vi "deeplabv3_onnx_camera.vi"() -> ()   [LabVIEW 2018]
uses:
  <vilib>/addons/VIRobotics/opencv_yiku/ctls/ColorConversionCodes.ctl
  <vilib>/addons/VIRobotics/opencv_yiku/Mat/Mat_32F/Mat_32F.lvclass
  C:/Program Files/National Instruments/LabVIEW 2018/vi.lib/addons/VIRobotics/opencv_yiku/Mat/Mat/Mat.lvclass
  <vilib>/addons/VIRobotics/opencv_yiku/Mat/Mat_8U/Mat_8U.lvclass
  <vilib>/addons/VIRobotics/opencv_yiku/Mat/Mat/Mat_length.vi
  <vilib>/addons/VIRobotics/onnx/Session/Get_Result_float.vi
  <vilib>/addons/VIRobotics/opencv_yiku/Mat/Mat/Mat_release.vi
  <vilib>/addons/VIRobotics/opencv_yiku/opencv_yiku.lvlib
  <vilib>/addons/VIRobotics/opencv_yiku/Mat/Mat/Mat.lvclass
  <vilib>/addons/VIRobotics/onnx/Session/Session.lvclass
  <vilib>/addons/VIRobotics/opencv_yiku/Cap/Cap.lvclass
panel:
  out "x-y":u32
  out "classes":cluster{"Color":u32, "name":string}[](array[cluster])
  in  "type":enum16{"CPU", "CUDA", "TensorRT"}(ring)=enum."TensorRT"
  in  "stop":bool
  out "mask":picture
  out "原始图像":picture
  out "合成的图像":picture
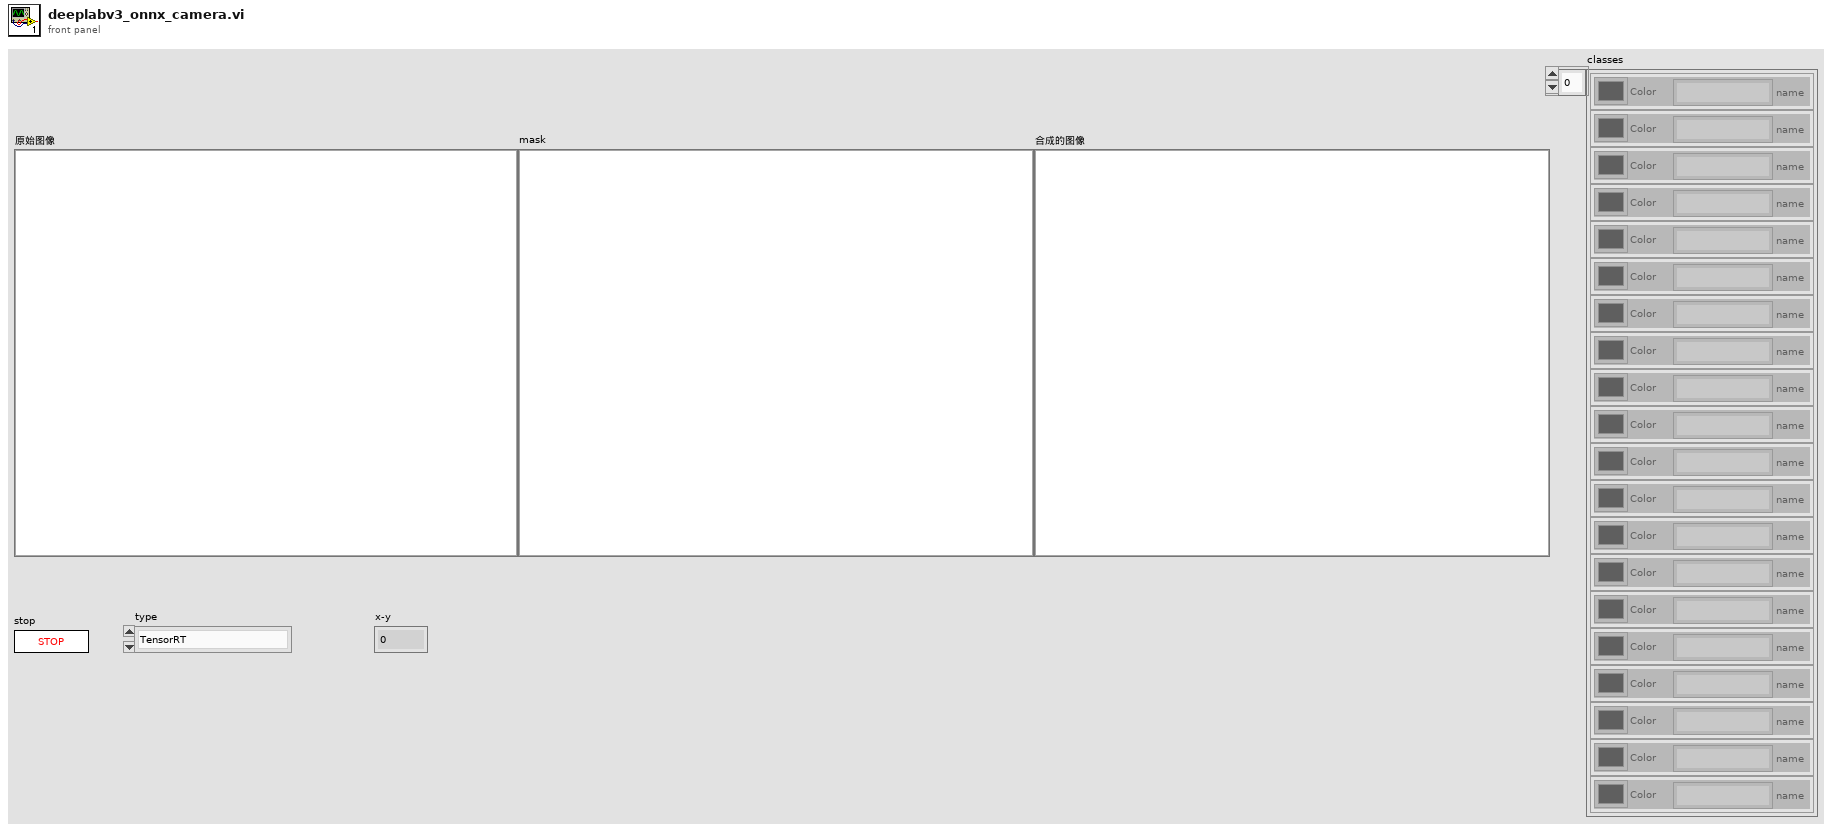
[diagram p1: front panel]
types:
  T1 = typedef "opencv_yiku.lvlib/ColorConversionCodes.ctl" = enum32{"COLOR_BGR2BGRA", "COLOR_BGRA2BGR", "COLOR_BGR2RGBA", "COLOR_RGBA2BGR", "COLOR_BGR2RGB", "COLOR_BGRA2RGBA", "COLOR_BGR2GRAY", "COLOR_RGB2GRAY", "COLOR_GRAY2BGR", "COLOR_GRAY2BGRA", "COLOR_BGRA2GRAY", "COLOR_RGBA2GRAY", "COLOR_BGR2BGR565", "COLOR_RGB2BGR565", "COLOR_BGR5652BGR", "COLOR_BGR5652RGB", "COLOR_BGRA2BGR565", "COLOR_RGBA2BGR565", "COLOR_BGR5652BGRA", "COLOR_BGR5652RGBA", "COLOR_GRAY2BGR565", "COLOR_BGR5652GRAY", "COLOR_BGR2BGR555", "COLOR_RGB2BGR555", "COLOR_BGR5552BGR", "COLOR_BGR5552RGB", "COLOR_BGRA2BGR555", "COLOR_RGBA2BGR555", "COLOR_BGR5552BGRA", "COLOR_BGR5552RGBA", "COLOR_GRAY2BGR555", "COLOR_BGR5552GRAY", "COLOR_BGR2XYZ", "COLOR_RGB2XYZ", "COLOR_XYZ2BGR", "COLOR_XYZ2RGB", "COLOR_BGR2YCrCb", "COLOR_RGB2YCrCb", "COLOR_YCrCb2BGR", "COLOR_YCrCb2RGB", "COLOR_BGR2HSV", "COLOR_RGB2HSV", "42", "43", "COLOR_BGR2Lab", "COLOR_RGB2Lab"}
  T2 = cluster{"height":i32, "width":i32, "channels":i32, "pointer":u64}
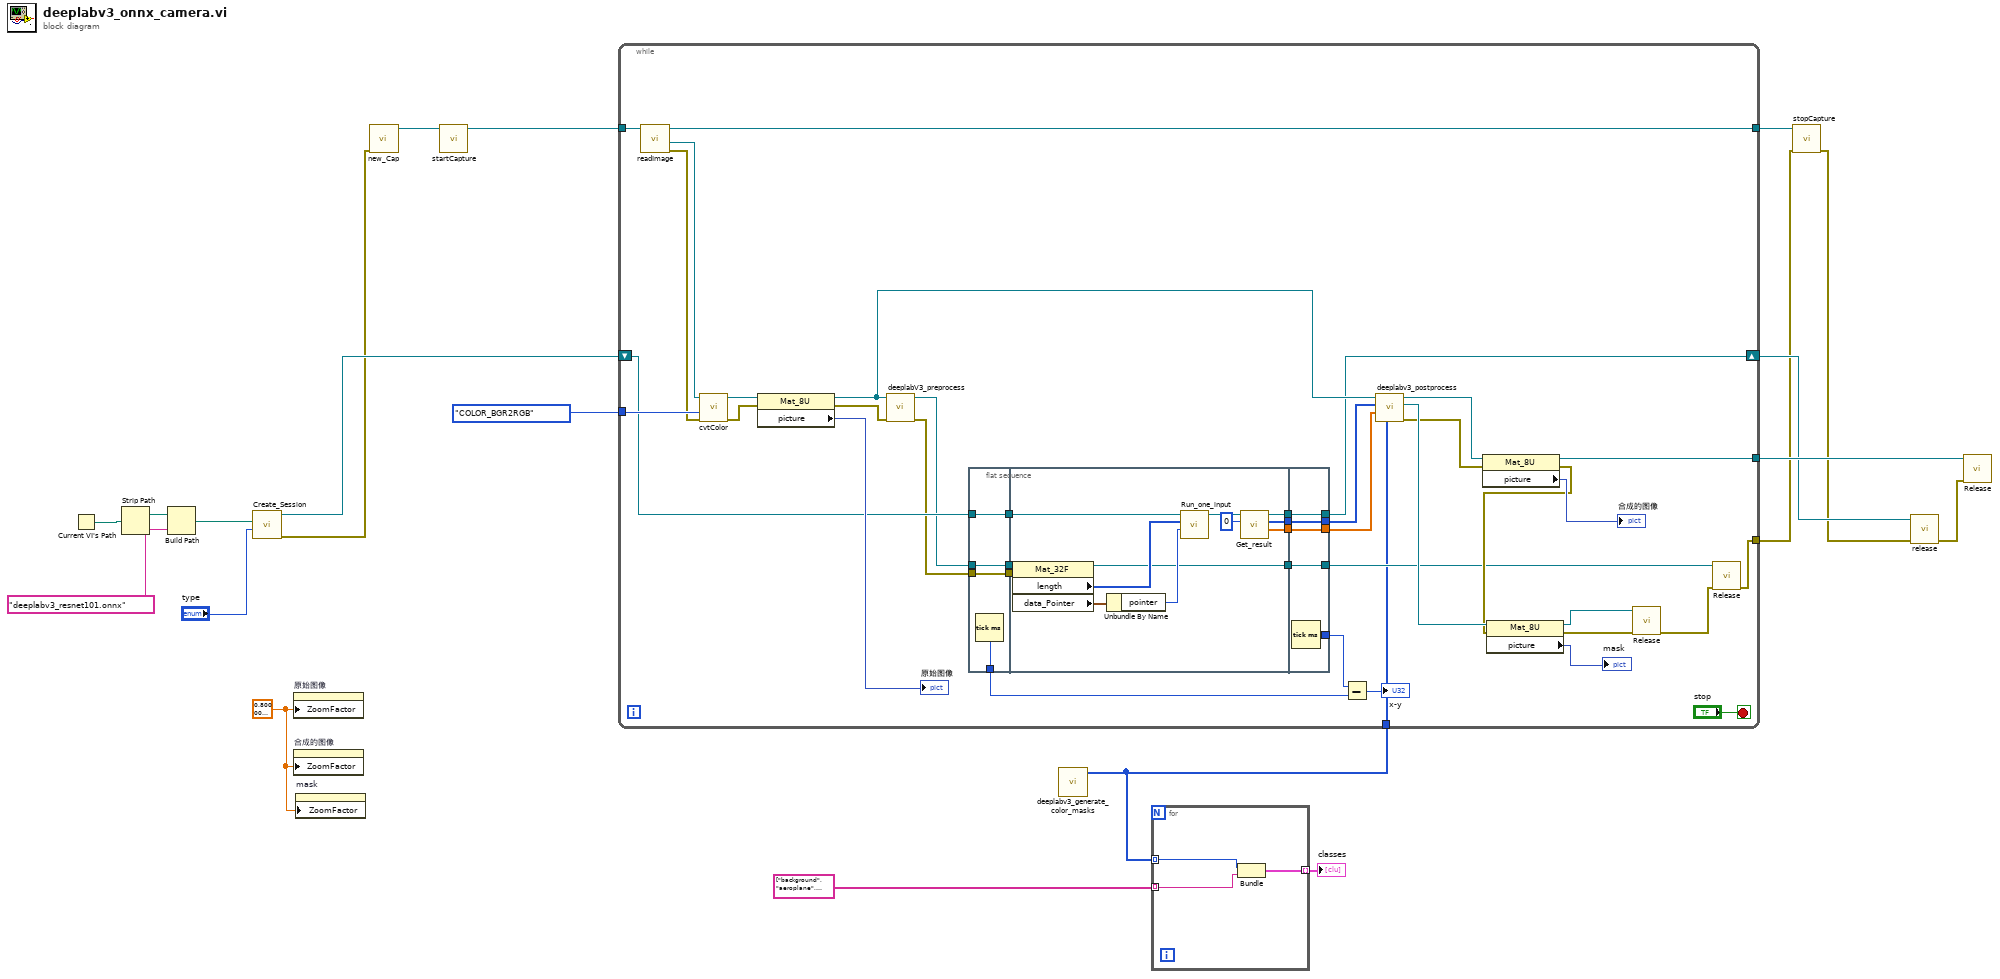
[diagram p0: block diagram]
diagram:
  w15 = sgl 0.8 ("Zoom Factor")
  n1 = Current VI's Path() -> (path=w19:path)
  n2 = Strip Path(path=w19) -> (stripped path=w20:path)  [unwired: 1 out]
  n3 = Build Path(base path=w20, name or relative path="deeplabv3_resnet101.onnx") -> (appended path=w13:path)
  n4 = call <vilib>:"Create_Session.vi"("type"="type", "path"=w13) -> ("error out"=w7:errorcluster, "Session out"=w12:refnum<class "Session.lvclass">)  [unwired: 8 in]
  n5 = property on="原始图像" class="Pict"("ZoomFactor"=w15) -> ()  [unwired: 2 in, 2 out]
  n6 = property on="合成的图像" class="Pict"("ZoomFactor"=w15) -> ()  [unwired: 2 in, 2 out]
  n7 = property on="mask" class="Pict"("ZoomFactor"=w15) -> ()  [unwired: 2 in, 2 out]
  n8 = call <vilib>:"new_Cap.vi"("error in (no error)"=w7) -> ("Cap out"=w9:refnum<class "Cap.lvclass">)  [unwired: 9 in, 1 out]
  n9 = call <vilib>:"startCapture.vi"("Cap in"=w9) -> ("Cap out"=w8:refnum<class "Cap.lvclass">)  [unwired: 9 in, 1 out]
  n10 = call "deeplabv3_generate_color_masks.vi"() -> ("colors"=w2:u32[])  [unwired: 11 in]
  n11 = while {
    tunnel: ColorConversionCodes."COLOR_BGR2RGB" ("dstCn") -> [w60]
    tunnel: [w55] -> w16
    shift-right: [w42] -> w10
    shift-left: w12 -> [w47]
    tunnel: w8 -> [w40]
    tunnel: [w37] -> w6
    tunnel: [w35] -> w5
    tunnel: w2 -> [w34]
    stop <- "stop" stop-if-true
    n12 = call <vilib>:"readImage.vi"("Cap in"=w40) -> ("error out"=w39:errorcluster, "Mat out"=w38:refnum<class "Mat_8U.lvclass">, "Cap out"=w37:refnum<class "Cap.lvclass">)  [unwired: 8 in]
    n13 = call <vilib>:"cvtColor.vi"("error in (no error)"=w39, "dstCn"=w60, "src"=w38) -> ("error out"=w53:errorcluster, "src out"=w59:refnum<class "Mat_8U.lvclass">)  [unwired: 6 in, 1 out]
    n14 = property class="Mat_8U"(reference=w59, error in=w53) -> (reference out=w52:refnum<class "Mat_8U.lvclass">, error out=w54:errorcluster, "picture"=→"原始图像":picture)
    n15 = call "deeplabV3_preprocess.vi"("error in (no error)"=w54, "img"=w52) -> ("error out"=w46:errorcluster, "blob"=w45:refnum<class "Mat_32F.lvclass">)  [unwired: 8 in]
    n16 = flat-sequence {
      tunnel: w45 -> [w62]
      tunnel: w46 -> [w63]
      tunnel: w47 -> [w64]
      tunnel: [w64] -> w26
      tunnel: [w63] -> w25
      tunnel: [w62] -> w24
      tunnel: [w61] -> w22
      tunnel: [w68] -> w30
      tunnel: [w67] -> w29
      tunnel: [w66] -> w28
      tunnel: [w65] -> w27
      tunnel: w26 -> [w76]
      tunnel: w25 -> [w75]
      tunnel: w24 -> [w74]
      tunnel: [w78] -> w36
      tunnel: [w79] -> w42
      tunnel: [w80] -> w43
      tunnel: [w81] -> w44
      tunnel: w30 -> [w81]
      tunnel: w29 -> [w80]
      tunnel: w28 -> [w79]
      tunnel: w27 -> [w78]
      tunnel: [w77] -> w23
      frame #0 {
        n17 = Tick Count (ms)() -> (millisecond timer value=w61:u32)
      }
      frame #1 {
        n18 = property class="Mat_32F"(reference=w74, error in=w75) -> (reference out=w65:refnum<class "Mat_32F.lvclass">, "length"=w73:i32[], "data_Pointer"=w72:T2)  [unwired: 1 out]
        n19 = Unbundle By Name(w72) -> ("pointer"=w71:u64)
        n20 = call <vilib>:"Run_one_input.vi"("data_pointer"=w71, "shape"=w73, "Session in"=w76) -> ("Session out"=w70:refnum<class "Session.lvclass">)  [unwired: 6 in, 2 out]
        n21 = call-poly <vilib>:"Get_result.vi"("index"=0, "Session in"=w70) -> ("data"=w67:sgl[], "shape"=w68:i64[], "Session out"=w66:refnum<class "Session.lvclass">)  [unwired: 6 in, 1 out]
      }
      frame #2 {
        n22 = Tick Count (ms)() -> (millisecond timer value=w77:u32)
      }
    }
    n23 = Subtract(x=w23, y=w22) -> (x-y=→"x-y":u32)
    n24 = call "deeplabv3_postprocess.vi"("colors"=w34, "1d_data"=w43, "length"=w44, "img in"=w52) -> ("error out"=w49:errorcluster, "mask"=w51:refnum<class "Mat_8U.lvclass">, "img out"=w57:refnum<class "Mat_8U.lvclass">)  [unwired: 5 in]
    n25 = property class="Mat_8U"(reference=w57, error in=w49) -> (reference out=w55:refnum<class "Mat_8U.lvclass">, error out=w48:errorcluster, "picture"=→"合成的图像":picture)
    n26 = property class="Mat_8U"(reference=w51, error in=w48) -> (reference out=w33:refnum<class "Mat_8U.lvclass">, error out=w32:errorcluster, "picture"=→"mask":picture)
    n27 = call-poly <vilib>:"Release.vi"("error in (no error)"=w32, "Mat in"=w33) -> ("error out"=w31:errorcluster)  [unwired: 9 in]
    n28 = call-poly <vilib>:"Release.vi"("error in (no error)"=w31, "Mat in"=w36) -> ("error out"=w35:errorcluster)  [unwired: 9 in]
  }
  n29 = for {
    tunnel: string[] ["background", "aeroplane", "bicycle", "bird", "boat", "bottle", "bus", "car", "cat", "chair", "cow", "diningtable", "dog", "horse", "motorbike", "person", "pottedplant", "sheep", "sofa", "train", "tvmonitor"] ("Array") -> [w83] mode=indexing
    tunnel: w2 -> [w84] mode=indexing
    tunnel: [w82] -> w1 mode=indexing
    n30 = Bundle("Color"=w84, "String"=w83) -> (w82:cluster{"Color":u32, "String":string})  [unwired: 1 in]
  }
  "classes" <- w1
  n31 = call <vilib>:"stopCapture.vi"("error in (no error)"=w5, "Cap in"=w6) -> ("error out"=w4:errorcluster)  [unwired: 9 in]
  n32 = call <vilib>:"release.vi"("error in (no error)"=w4, "Session in"=w10) -> ("error out"=w11:errorcluster)  [unwired: 9 in]
  n33 = call-poly <vilib>:"Release.vi"("error in (no error)"=w11, "Mat in"=w16) -> ()  [unwired: 9 in, 1 out]
